vi "DeviceInitialize.vi"(8 "error in (no error)":errorcluster, 9 "Reset (True)":bool=TRUE, 10 "ID Query (True)":bool=TRUE, 11 "TesteractHAL_DigitalOutput_EthernetModbus In":refnum<class "TesteractHAL_DigitalOutput_EthernetModbus.lvclass">) -> (0 "error out":errorcluster, 3 "TesteractHAL_DigitalOutput_EthernetModbus Out":refnum<class "TesteractHAL_DigitalOutput_EthernetModbus.lvclass">)   [LabVIEW 2017, in "TesteractHAL_DigitalOutput_EthernetModbus.lvlib" / "TesteractHAL_DigitalOutput_EthernetModbus.lvclass"]
uses:
  TesteractHAL_DigitalOutput_EthernetModbus.lvclass
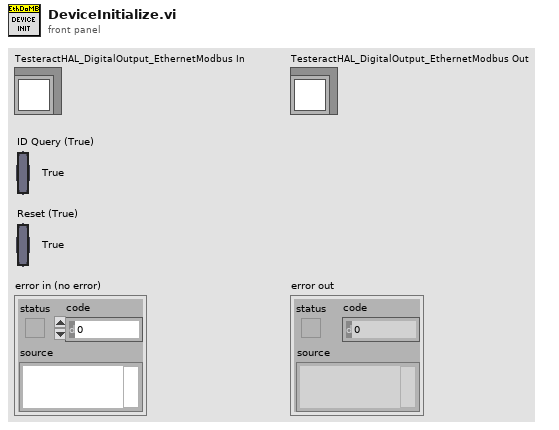
[diagram p1: front panel]
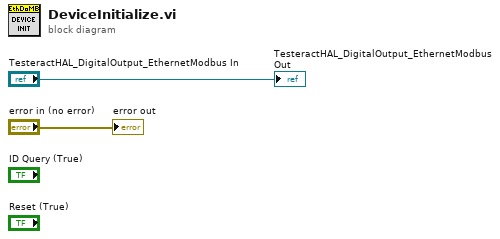
[diagram p0: block diagram]
diagram:
  "error out" <- "error in (no error)"
  "TesteractHAL_DigitalOutput_EthernetModbus Out" <- "TesteractHAL_DigitalOutput_EthernetModbus In"
